vi "File Exists.vi"(11 "Path":path) -> (1 "Is Directory?":bool, 3 "Exists?":bool)   [LabVIEW 2023]
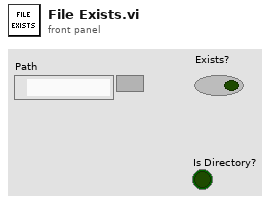
[diagram p1: front panel]
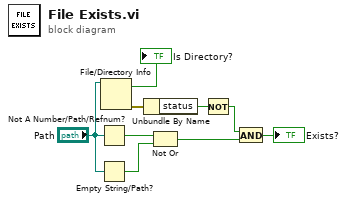
[diagram p0: block diagram]
diagram:
  n1 = Not A Number/Path/Refnum?(number/path/refnum="Path") -> (NaN/Path/Refnum?=w4:bool)
  n2 = Empty String/Path?(string/path="Path") -> (empty?=w3:bool)
  n3 = File/Directory Info(path="Path") -> (directory=→"Is Directory?":bool, error out=w5:errorcluster)  [unwired: 1 in, 5 out]
  n4 = Unbundle By Name(w5) -> ("status"=w6:bool)
  n5 = Not Or(1:w3, 2:w4) -> (0:w9:bool)
  n6 = Not(x=w6) -> (.not. x?=w8:bool)
  n7 = And(x=w8, y=w9) -> (x .and. y?=→"Exists?":bool)
